vi "chirp_waitV3.vi"(8 "error in (no error)":errorcluster, 11 "ChirpV2 in":refnum<class "ChirpV2.lvclass">) -> (0 "error out":errorcluster, 2 "data":dynamicdata(graph), 3 "ChirpV2 out":refnum<class "ChirpV2.lvclass">)   [LabVIEW 2014, in "ChirpV2.lvclass"]
uses:
  ChirpV2.lvclass
  <vilib>/Analysis/4window.llb/Cosine Tapered Window (DBL).vi
  <vilib>/measure/NI_MABase.lvlib
  <vilib>/addons/_NISVFA/_Generation/SoundVib_Generation.lvlib
  <vilib>/Analysis/NI_AALPro.lvlib
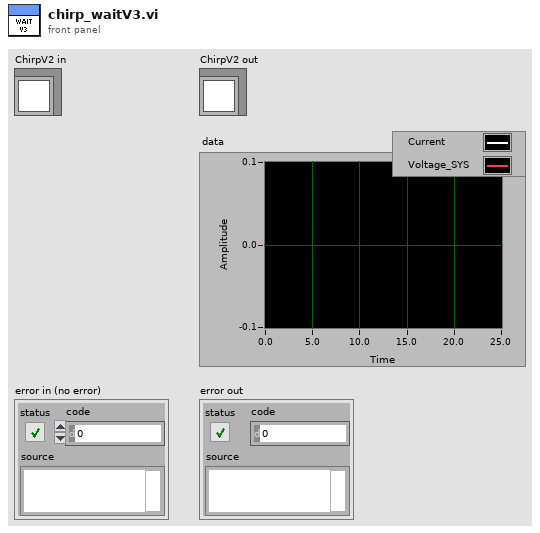
[diagram p1: front panel]
types:
  T1 = cluster{"start frequency [Hz]":dbl, "stop frequency [Hz]":dbl}
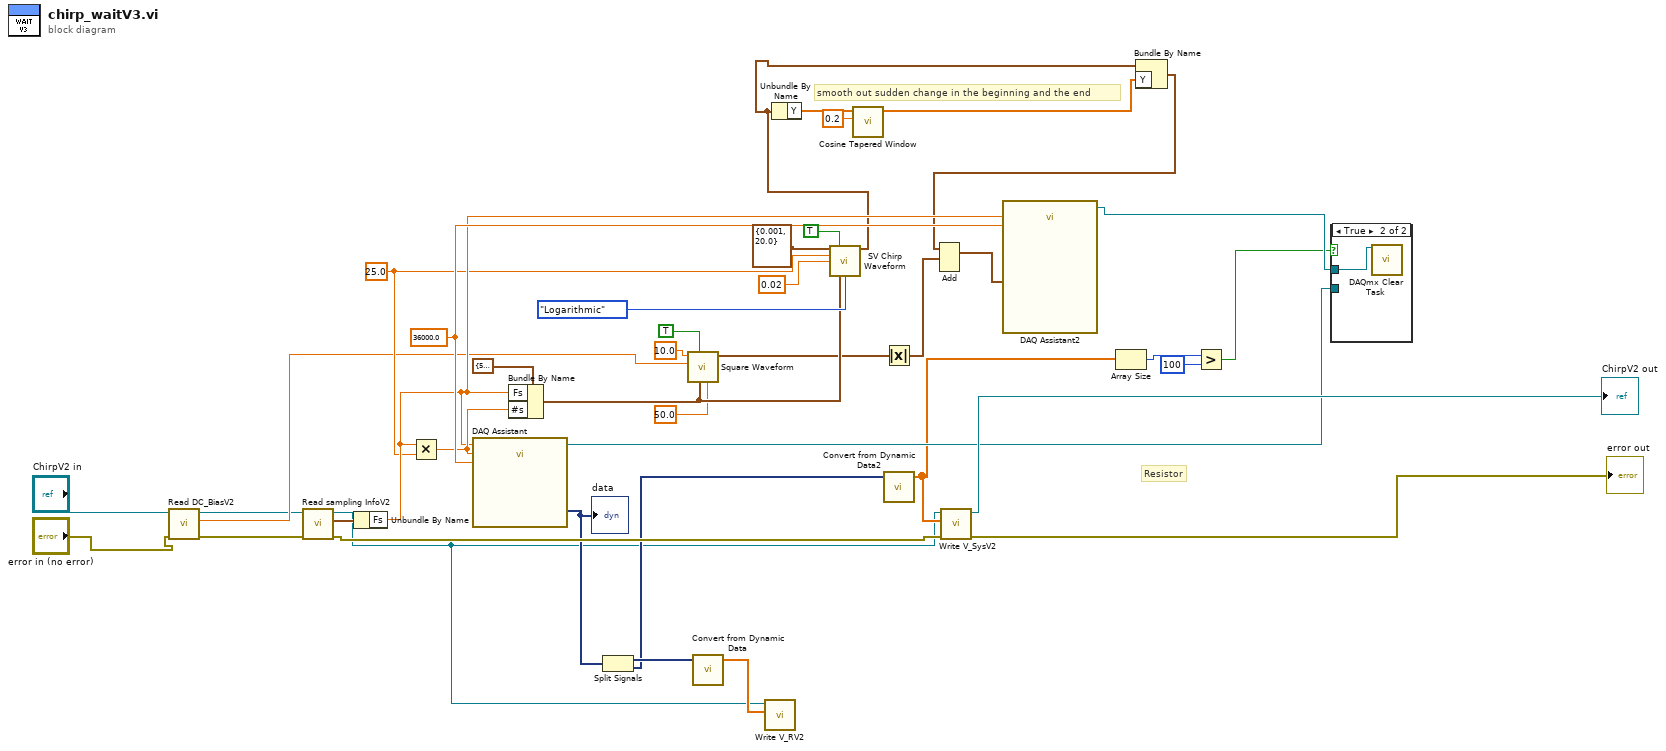
[diagram p0: block diagram]
diagram:
  w40 = 36000.0 ("timeout (s)")
  w35 = 25.0 ("y")
  # "smooth out sudden change in the beginning and the end"
  # "Resistor"
  n1 = call-dynamic "Read DC_BiasV2.vi"("error in (no error)"="error in (no error)", "ChirpV2 in"="ChirpV2 in") -> ("error out"=w26:errorcluster, "DC_Bias"=w27:dbl, "ChirpV2 out"=w25:refnum<class "ChirpV2.lvclass">)  [unwired: 7 in]
  n2 = call-dynamic "Read sampling InfoV2.vi"("error in (no error)"=w26, "ChirpV2 in"=w25) -> ("error out"=w6:errorcluster, "sampling Info"=w28:cluster{"Fs":dbl}, "ChirpV2 out"=w1:refnum<class "ChirpV2.lvclass">)  [unwired: 7 in]
  n3 = Unbundle By Name(w28) -> ("Fs"=w38:dbl)
  n4 = Multiply(x=w38, y=w35) -> (x*y=w39:dbl)
  n5 = call "DAQ Assistant"("rate"=w38, "number of samples"=w39, "timeout (s)"=w40) -> ("task out"=w12:refnum<k21>, "data"=w3:dynamicdata)  [unwired: 14 in, 1 out]
  "data" <- w3
  n6 = Bundle By Name(cluster=cluster{"Fs":dbl, "#s":u32} {"Fs"=51200.0, "#s"=1024} ("sampling info"), "Fs"=w38, "#s"=w39) -> (w30:cluster{"Fs":dbl, "#s":u32})
  n7 = Split Signals(w3) -> (w4:dynamicdata, w2:dynamicdata)  [unwired: 2 in]
  n8 = call <vilib>:"Square Waveform.vi"("duty cycle (%)"=50.0, "sampling info"=w30, "reset signal"=TRUE, "amplitude"=w27, "frequency"=10.0) -> ("signal out"=w23:waveform(dbl))  [unwired: 5 in, 1 out]
  n9 = call "Convert from Dynamic Data"("Dynamic Data Type"=w4) -> ("Array"=w5:dbl[])  [unwired: 3 in]
  n10 = call-dynamic "Write V_RV2.vi"("V_R"=w5, "ChirpV2 in"=w1) -> ()  [unwired: 8 in, 2 out]
  n11 = call <vilib>:"SV Chirp Waveform.vi"("frequency range"=T1 {"start frequency [Hz]"=0.001, "stop frequency [Hz]"=20.0}, "reset signal (F)"=TRUE, "chirp duration [s]"=w35, "amplitude"=0.02, "sampling info"=w30, "frequency spacing"=enum16{"Linear", "Logarithmic"}."Logarithmic") -> ("chirp signal"=w17:waveform(dbl))  [unwired: 7 in, 2 out]
  n12 = Unbundle By Name(w17) -> ("Y"=w18:dbl[])
  n13 = call-poly <vilib>:"Cosine Tapered Window.vi"("ratio"=0.2, "X"=w18) -> ("Windowed X"=w19:dbl[])  [unwired: 8 in, 1 out]
  n14 = Absolute Value(x=w23) -> (abs(x)=w32:waveform(dbl))
  n15 = call "Convert from Dynamic Data2"("Dynamic Data Type"=w2) -> ("Array"=w10:dbl[])  [unwired: 3 in]
  n16 = call-dynamic "Write V_SysV2.vi"("error in (no error)"=w6, "V_Sys"=w10, "ChirpV2 in"=w1) -> ("error out"=→"error out":errorcluster, "ChirpV2 out"=→"ChirpV2 out":refnum<class "ChirpV2.lvclass">)  [unwired: 7 in]
  n17 = Array Size(array=w10) -> (size(s)=w9:i32)
  n18 = Bundle By Name(cluster=w17, "Y"=w19) -> (w16:waveform(dbl))
  n19 = Add(1:w32, 2:w16) -> (0:w34:waveform(dbl))  [unwired: 1 in, 1 out]
  n20 = call "DAQ Assistant2"("data"=w34, "rate"=w38, "timeout (s)"=w40) -> ("task out"=w13:refnum<k21>)  [unwired: 14 in, 2 out]
  n21 = Greater?(x=w9, y=100) -> (0:w8:bool)
  n22 = case shown="True" w8 {
    tunnel: w12 -> [_ _]
    tunnel: w13 -> [_ w42]
    frame False {
    }
    frame True {
      n23 = call <vilib>:"DAQmx Clear Task.vi"("task in"=w42) -> ()  [unwired: 14 in, 1 out]
    }
  }
